vi "ListVIsOfMethod.vi"(1 "VI Refnum":refnum<vi>, 5 "error in (no error)":errorcluster) -> (15 "Refs":refnum<vi>[](array[refnum]), 16 "Names":string[](array[string]), 19 "error out":errorcluster)   [LabVIEW 2013]
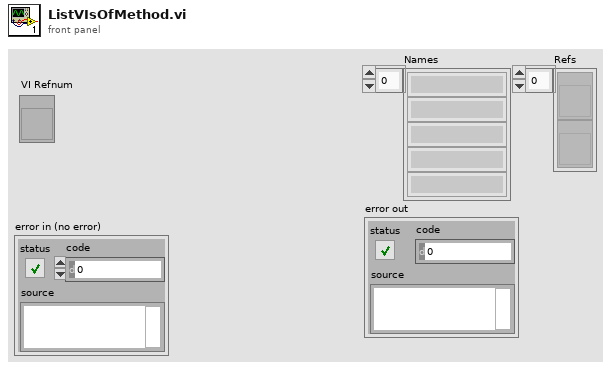
[diagram p1: front panel]
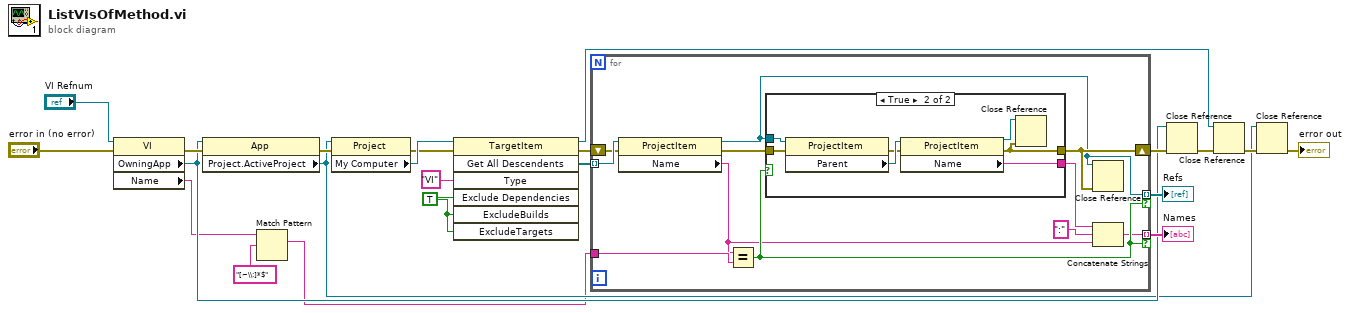
[diagram p0: block diagram]
diagram:
  w21 = TRUE ("ExcludeDependencies")
  n1 = property class="VI"(reference="VI Refnum", error in="error in (no error)") -> (error out=w15:errorcluster, "OwningApp"=w9:refnum<vi>, "Name"=w2:string)  [unwired: 1 out]
  n2 = property class="App"(reference=w9, error in=w15) -> (error out=w14:errorcluster, "Project.ActiveProject"=w5:refnum<vi>)  [unwired: 1 out]
  n3 = Match Pattern(string=w2, regular expression="[~\\:]*$") -> (match substring=w1:string)  [unwired: 4 out]
  n4 = property class="Project"(reference=w5, error in=w14) -> (error out=w13:errorcluster, "My Computer"=w22:refnum<vi>)  [unwired: 1 out]
  n5 = invoke class="TargetItem" method="Get All Descendents"(reference=w22, error in=w13, "Type"="VI", "Exclude Dependencies"=w21, "ExcludeBuilds"=w21, "ExcludeTargets"=w21) -> (reference out=w7:refnum<vi>, error out=w12:errorcluster, "All Descendents"=w19:refnum<vi>[])  [unwired: 1 in, 4 out]
  n6 = for {
    tunnel: w19 -> [w33] mode=indexing
    tunnel: [w25] -> w18 mode=indexing if=w30
    tunnel: w1 -> [w32]
    tunnel: [w23] -> w17 mode=indexing if=w30
    shift-right: [w24] -> w10
    shift-left: w12 -> [w31]
    n7 = property class="ProjectItem"(reference=w33, error in=w31) -> (reference out=w23:refnum<vi>, error out=w29:errorcluster, "Name"=w26:string)
    n8 = Equal?(x=w26, y=w32) -> (x = y?=w30:bool)
    n9 = case shown="True" w30 {
      tunnel: w29 -> [w34 w41]
      tunnel: w23 -> [_ w40]
      tunnel: [_ w37] -> w28
      tunnel: [w34 w35] -> w24
      frame False {
      }
      frame True {
        n10 = property class="ProjectItem"(reference=w40, error in=w41) -> (error out=w36:errorcluster, "Parent"=w39:refnum<vi>)  [unwired: 1 out]
        n11 = property class="ProjectItem"(reference=w39, error in=w36) -> (reference out=w38:refnum<vi>, error out=w35:errorcluster, "Name"=w37:string)
        n12 = Close Reference(reference=w38, error in (no error)=w35) -> ()  [unwired: 1 out]
      }
    }
    n13 = Close Reference(reference=w23, error in (no error)=w24) -> ()  [unwired: 1 out]
    n14 = Concatenate Strings(w28, ":" ("string"), w26) -> (w25:string)
  }
  "Names" <- w18
  "Refs" <- w17
  n15 = Close Reference(reference=w9, error in (no error)=w10) -> (error out=w8:errorcluster)
  n16 = Close Reference(reference=w7, error in (no error)=w8) -> (error out=w6:errorcluster)
  n17 = Close Reference(reference=w5, error in (no error)=w6) -> (error out=→"error out":errorcluster)
